vi "Configure.vi"(8 "error in (no error)":errorcluster, 11 "Tomo in":refnum<class "Tomo.lvclass">) -> (0 "error out":errorcluster, 2 "cancelled?":bool, 3 "Tomo out":refnum<class "Tomo.lvclass">)   [LabVIEW 2012, in "Tomo.lvclass"]
doc: "The configure method configures the details for the RabbitMQ connection. \n\nIn the derived class, make a call to the parent for setting these parameters."
uses:
  Tomo.lvclass
  <vilib>/Utility/miscctls.llb/LVPointTypeDef.ctl
  Tomo.lvclass/Tomo.ctl
  <vilib>/Distrio/Murmex/Murmex/Murmex.lvclass
panel:
  in  "Tab Control":enum32{"Slave components", "Others", "Pre-tomo"}(tab)
  in  "pretomo camera component":string
  in  "imaging component":string
  in  "stack component":string
  in  "camera component":string
  in  "stages component":string
  in  "autofocus component":string
  in  "AOTF component":string
  in  "mapping file folder":path
  in  "default stages speed":dbl[unit]
  in  "stack overhead time":dbl[unit]
  in  "camera pixel size":dbl[unit]=0.00039999999999999996
  in  "Y step size":dbl[unit]=0.00039999999999999996
  in  "X step size":dbl[unit]=0.00039999999999999996
  in  "Z step size":dbl[unit]=2e-06
  in  "downsampling factor":u32
  in  "camera y res":u32
  in  "camera x res":u32
  in  "small images base path":path
  in  "full image base path":path
  in  "button::cancel":bool
  in  "button::configure_murmex":bool
  in  "button::ok":bool
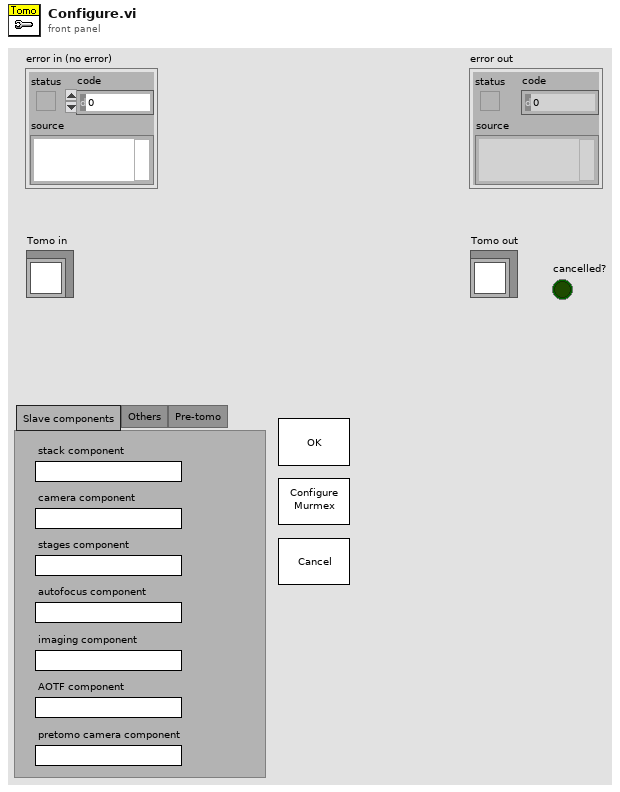
[diagram p1: front panel]
types:
  T1 = typedef "LVPointTypeDef.ctl" = cluster{"Horizontal":i16, "Vertical":i16}
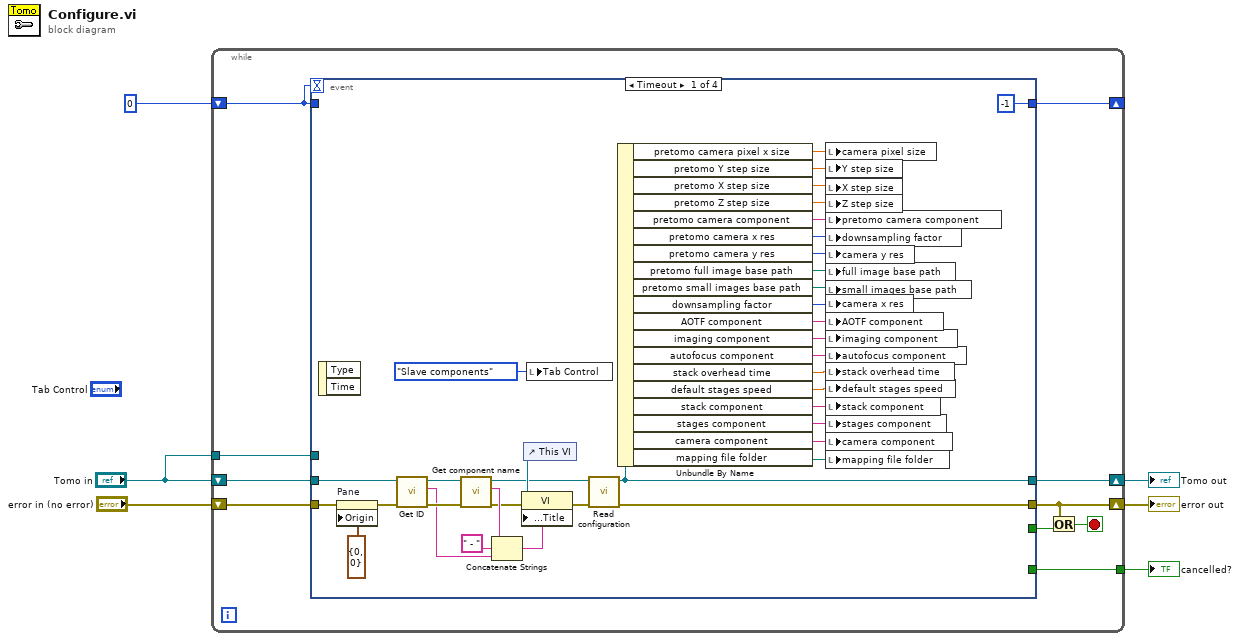
[diagram p0: block diagram]
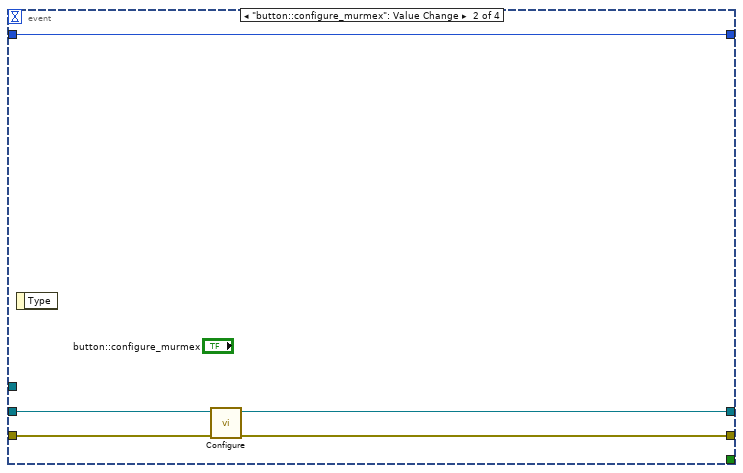
[diagram p2: hidden frame]
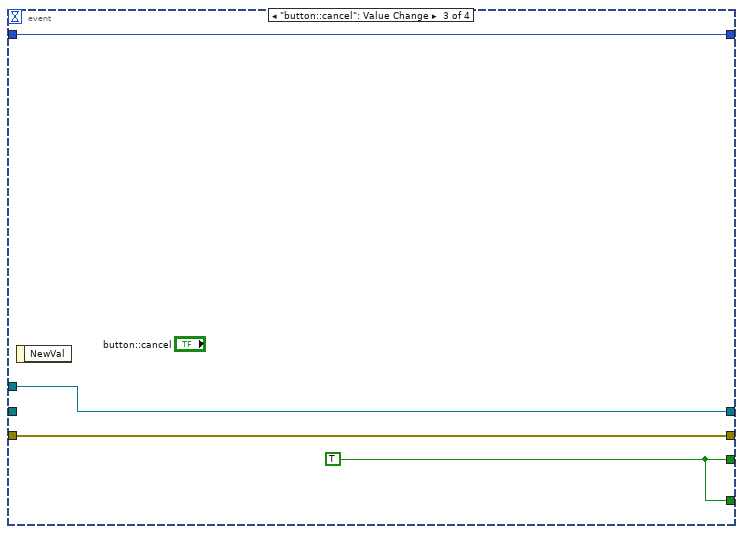
[diagram p3: hidden frame]
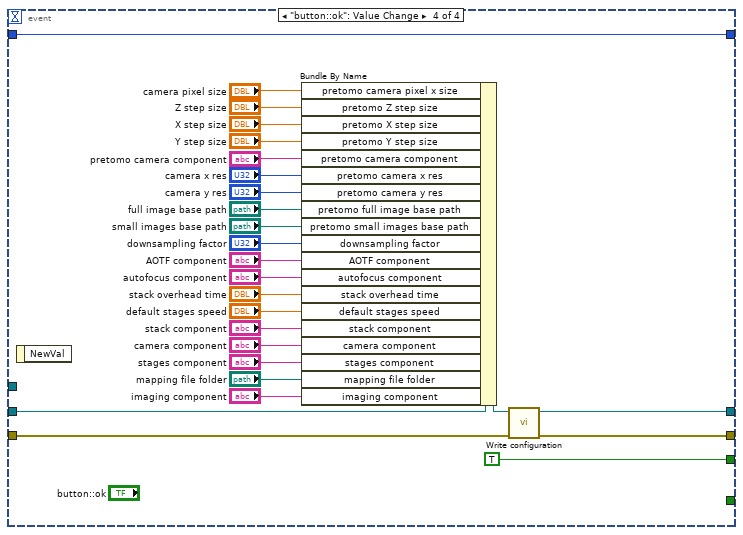
[diagram p4: hidden frame]
diagram:
  n1 = while {
    shift-right: [w9] -> w2
    shift-left: "error in (no error)" -> [w16]
    shift-right: [w12] -> _
    shift-left: 0 -> [w15]
    shift-right: [w11] -> w1
    shift-left: "Tomo in" -> [w14]
    tunnel: "Tomo in" -> [w13]
    tunnel: [w7] -> w3
    stop <- w8 stop-if-true
    n2 = event shown="[0] Timeout" {
      selector: _ -> [_ _ _ _]
      dyn-events: _ -> [_ _ _ _]
      timeout: w15 -> [_ _ _ _]
      tunnel: w16 -> [w53 w58 w61 w84]
      tunnel: w15 -> [_ w54 w59 w88]
      tunnel: w14 -> [w50 w56 _ w83]
      tunnel: w13 -> [_ _ w62 _]
      tunnel: [-1 w54 w59 w88] -> w12
      tunnel: [w37 w55 w62 w85] -> w11
      tunnel: [w38 w57 w61 w87] -> w9
      tunnel: [_ _ w60 TRUE] -> w10
      tunnel: [_ _ w60 _] -> w7
      event Timeout {
        n3 = event-data() -> ()  [unwired: 1 in, 2 out]
        n4 = property on="Pane" class="Pane"(error in=w53, "Origin"=T1 {"Horizontal"=0, "Vertical"=0}) -> (error out=w51:errorcluster)  [unwired: 1 in, 1 out]
        n5 = call <vilib>:"Get ID.vi"("error in (no error)"=w51, "Murmex in"=w50) -> ("error out"=w49:errorcluster, "component id"=w46:string, "Murmex out"=w48:refnum<class "Tomo.lvclass">)  [unwired: 7 in]
        n6 = call <vilib>:"Get component name.vi"("error in (no error)"=w49, "Murmex in"=w48) -> ("error out"=w43:errorcluster, "component name"=w47:string, "Murmex out"=w39:refnum<class "Tomo.lvclass">)  [unwired: 7 in]
        n7 = Concatenate Strings(w47, " - " ("string"), w46) -> (w41:string)
        n8 = control-ref of="This VI"() -> (w42:refnum<vi>)
        n9 = property class="VI"(reference=w42, error in=w43, "Front Panel.Title"=w41) -> (error out=w40:errorcluster)  [unwired: 1 out]
        n10 = local write "Tab Control"(enum32{"Slave components", "Others"}."Slave components" ("Tab Control")) -> ()
        n11 = call <vilib>:"Read configuration.vi"("error in (no error)"=w40, "Murmex in"=w39) -> ("error out"=w38:errorcluster, "Murmex out"=w37:refnum<class "Tomo.lvclass">)  [unwired: 7 in, 1 out]
        n12 = Unbundle By Name(w37) -> ("pretomo camera pixel x size"=w17:dbl[unit], "pretomo Y step size"=w18:dbl[unit], "pretomo X step size"=w19:dbl[unit], "pretomo Z step size"=w20:dbl[unit], "pretomo camera component"=w21:string, "pretomo camera x res"=w23:u32, "pretomo camera y res"=w24:u32, "pretomo full image base path"=w26:path, "pretomo small images base path"=w25:path, "downsampling factor"=w22:u32, "AOTF component"=w27:string, "imaging component"=w28:string, "autofocus component"=w30:string, "stack overhead time"=w32:dbl[unit], "default stages speed"=w31:dbl[unit], "stack component"=w33:string, "stages component"=w34:string, "camera component"=w35:string, "mapping file folder"=w36:path)
        n13 = local write "camera pixel size"(w17) -> ()
        n14 = local write "Y step size"(w18) -> ()
        n15 = local write "X step size"(w19) -> ()
        n16 = local write "Z step size"(w20) -> ()
        n17 = local write "pretomo camera component"(w21) -> ()
        n18 = local write "downsampling factor"(w23) -> ()
        n19 = local write "camera y res"(w24) -> ()
        n20 = local write "full image base path"(w26) -> ()
        n21 = local write "small images base path"(w25) -> ()
        n22 = local write "camera x res"(w22) -> ()
        n23 = local write "AOTF component"(w27) -> ()
        n24 = local write "imaging component"(w28) -> ()
        n25 = local write "autofocus component"(w30) -> ()
        n26 = local write "stack overhead time"(w32) -> ()
        n27 = local write "default stages speed"(w31) -> ()
        n28 = local write "stack component"(w33) -> ()
        n29 = local write "stages component"(w34) -> ()
        n30 = local write "camera component"(w35) -> ()
        n31 = local write "mapping file folder"(w36) -> ()
      }
      event "button::configure_murmex": Value Change {
        n32 = event-data() -> ()  [unwired: 1 in, 1 out]
        n33 = call-parent "Configure.vi"("error in (no error)"=w58, "Murmex in"=w56) -> ("error out"=w57:errorcluster, "Murmex out"=w55:refnum<class "Tomo.lvclass">)  [unwired: 7 in, 1 out]
      }
      event "button::cancel": Value Change {
        w60 = TRUE
        n34 = event-data() -> ()  [unwired: 1 in, 1 out]
      }
      event "button::ok": Value Change {
        n35 = event-data() -> ()  [unwired: 1 in, 1 out]
        n36 = Bundle By Name(cluster=w83, "pretomo camera pixel x size"="camera pixel size", "pretomo Z step size"="Z step size", "pretomo X step size"="X step size", "pretomo Y step size"="Y step size", "pretomo camera component"="pretomo camera component", "pretomo camera x res"="camera x res", "pretomo camera y res"="camera y res", "pretomo full image base path"="full image base path", "pretomo small images base path"="small images base path", "downsampling factor"="downsampling factor", "AOTF component"="AOTF component", "autofocus component"="autofocus component", "stack overhead time"="stack overhead time", "default stages speed"="default stages speed", "stack component"="stack component", "camera component"="camera component", "stages component"="stages component", "mapping file folder"="mapping file folder", "imaging component"="imaging component") -> (w82:refnum<class "Tomo.lvclass">)
        n37 = call <vilib>:"Write configuration.vi"("error in (no error)"=w84, "Murmex in"=w82) -> ("error out"=w87:errorcluster, "Murmex out"=w85:refnum<class "Tomo.lvclass">)  [unwired: 8 in]
      }
    }
    n38 = Or(x=w9, y=w10) -> (x .or. y?=w8:bool)
  }
  "error out" <- w2
  "Tomo out" <- w1
  "cancelled?" <- w3
